vi "OCV_DMM_ApertureTime_StdDev.vi"() -> ()   [LabVIEW 2019]
panel:
  out "Error 6.5 digits AZon ADCCalon":dbl[](array[numeric])=[-1.2854850467647339e-05, -7.886710542415187e-06, 8.316335529112706e-06, 6.3393632019348445e-06, 8.358046865719615e-06] format="%#_7p"
  in  "mean values of channels 6.5 digits AZon ADCcal on":dbl[](array[numeric])=[3.4860065278089722, 3.48375553663424, 3.4808778023254034, 3.484652928409848, 3.4829310355717924] format="%#_7p"
  in  "Mean values of channels - shorted at Pogo Pins":dbl[](array[numeric])=[-6.355978921184258e-06, 2.501900814016391e-06, 1.0081969476181121e-05, 3.7724183553781954e-06, 5.872057669979462e-06] format="%#_7p"
  out "Error 100ms":dbl[](array[numeric])=[-9.674542087889648e-06, -1.2342180970570382e-06, 1.8209219958098544e-05, 4.237175472265875e-06, 4.739579464008159e-06] format="%#_7p"
  in  "Mean values of channels 100ms":dbl[](array[numeric])=[3.486009708117352, 3.4837621891266854, 3.4808876952098324, 3.4846508262221185, 3.4829274171043907] format="%#_7p"
  out "Error 83.3333ms":dbl[](array[numeric])=[-7.575016874206142e-06, -6.872566817861525e-07, 1.9622864356083625e-05, 6.5984626940185365e-06, 4.496907730189292e-06] format="%#_7p"
  in  "Mean values of channels 83.333ms":dbl[](array[numeric])=[3.4860118076425657, 3.4837627360881007, 3.4808891088542304, 3.4846531875093403, 3.482927174432657] format="%#_7p"
  out "Error 66.6666ms":dbl[](array[numeric])=[-9.609345659189472e-06, -2.0157464732939445e-06, 1.7317177337439205e-05, 4.952653229306492e-06, 4.43857256948732e-06] format="%#_7p"
  in  "Mean values of channels 66.666ms":dbl[](array[numeric])=[3.4860097733137807, 3.483761407598309, 3.4808868031672118, 3.4846515416998756, 3.482927116097496] format="%#_7p"
  out "Error 50ms":dbl[](array[numeric])=[-9.493969597151874e-06, -1.1936376171917118e-06, 1.7657588552655312e-05, 4.130477512909181e-06, 4.090088825403626e-06] format="%#_7p"
  in  "Mean values of channels 50ms":dbl[](array[numeric])=[3.4860098886898427, 3.4837622297071653, 3.480887143578427, 3.484650719524159, 3.482926767613752] format="%#_7p"
  out "Error 33.3333ms":dbl[](array[numeric])=[-9.17710259651372e-06, -2.6768859844317205e-06, 1.6583768505107344e-05, 4.873448069098174e-06, 3.1290639057601766e-06] format="%#_7p"
  in  "Mean values of channels 33.3333ms":dbl[](array[numeric])=[3.4860102055568434, 3.483760746458798, 3.4808860697583794, 3.4846514624947154, 3.4829258065888324] format="%#_7p"
  out "Error 16.6666ms":dbl[](array[numeric])=[-9.674542087889648e-06, -1.2342180970570382e-06, 1.8209219958098544e-05, 4.237175472265875e-06, 4.739579464008159e-06] format="%#_7p"
  in  "Mean values of channels 7.5 digits manual":dbl[](array[numeric])=[3.48601938265944, 3.4837634233447825, 3.4808694859898743, 3.4846465890466463, 3.4829226775249267] format="%#_7p"
  in  "Mean values of channels 16.6666ms":dbl[](array[numeric])=[3.486009708117352, 3.4837621891266854, 3.4808876952098324, 3.4846508262221185, 3.4829274171043907] format="%#_7p"
  in  "4":dbl=41.179 format="%#_6p"
  in  "3":dbl=5.212e-06 format="%#_6p"
  in  "2":dbl=1.52e-06 format="%#_6p"
  in  "1":dbl=0.2 format="%#_6p"
  in  "Test Time (s)":dbl[](array[numeric])=[4.463, 7.822, 11.163, 14.513, 17.84, 21.179] format="%#_6p"
  in  "Range (V)":dbl[](array[numeric])=[8.642e-06, 1.954e-06, 2.665e-06, 1.721e-06, 2.407e-06, 2.652e-06] format="%#_6p"
  in  "Standard Deviation (V)":dbl[](array[numeric])=[2.601e-06, 4.67064e-07, 7.14041e-07, 4.0509e-07, 6.56265e-07, 6.5863e-07] format="%#_6p"
  in  "DMM Aperture Time (s)":dbl[](array[numeric])=[0.0166666, 0.033333, 0.05, 0.0666666, 0.0833333, 0.1] format="%#_6p"
  in  "DMM Resolution (Digits)":dbl[](array[numeric])=[3.5, 4.5, 5.5, 6.5, 6.5, 7.5] format="%#_6p"
  in  "Range (V) Digits":dbl[](array[numeric])=[6.9339e-05, 7.3891e-05, 2.2514e-05, 3.346e-06, 5.505e-06, 8.62e-06] format="%#_6p"
  out "Standard Deviation vs Aperture Time":T1(graph)={"Standard Deviation (Ohm)"=[0.0166666, 0.033333, 0.05, 0.0666666, 0.0833333, 0.1], "Aperture Time (s)"=[2.601e-06, 4.67064e-07, 7.14041e-07, 4.0509e-07, 6.56265e-07, 6.5863e-07]}
  in  "Test Time (s) Digits":dbl[](array[numeric])=[1.317, 1.322, 1.418, 21.181, 57.59, 227.179] format="%#_6p"
  in  "Standard Deviation (V) Digits":dbl[](array[numeric])=[1.5947e-05, 1.7401e-05, 5.913e-06, 9.48824e-07, 1.534e-06, 2.201e-06] format="%#_6p"
  in  "DMM Aperture Time (s) Digits":dbl[](array[numeric])=[2e-05, 2e-05, 0.0005, 0.1, 0.1, 0.1] format="%#_6p"
  # "1 Average, AutoZero Once, ADC Cal Off, Settle Time 1ms"
  # "1 Average, AutoZero Once, ADC Cal Off, Settle Time 1ms"
  # "1 Average, AutoZero Once, ADC Cal Off, Settle Time 1ms"
  # "1 Average, AutoZero Once, ADC Cal Off, Settle Time 0ms"
  # "1 Average, AutoZero On, ADC Cal On, Settle Time 1ms"
  # "4 Averages, AutoZero On, ADC Cal On, Settle Time 1ms"
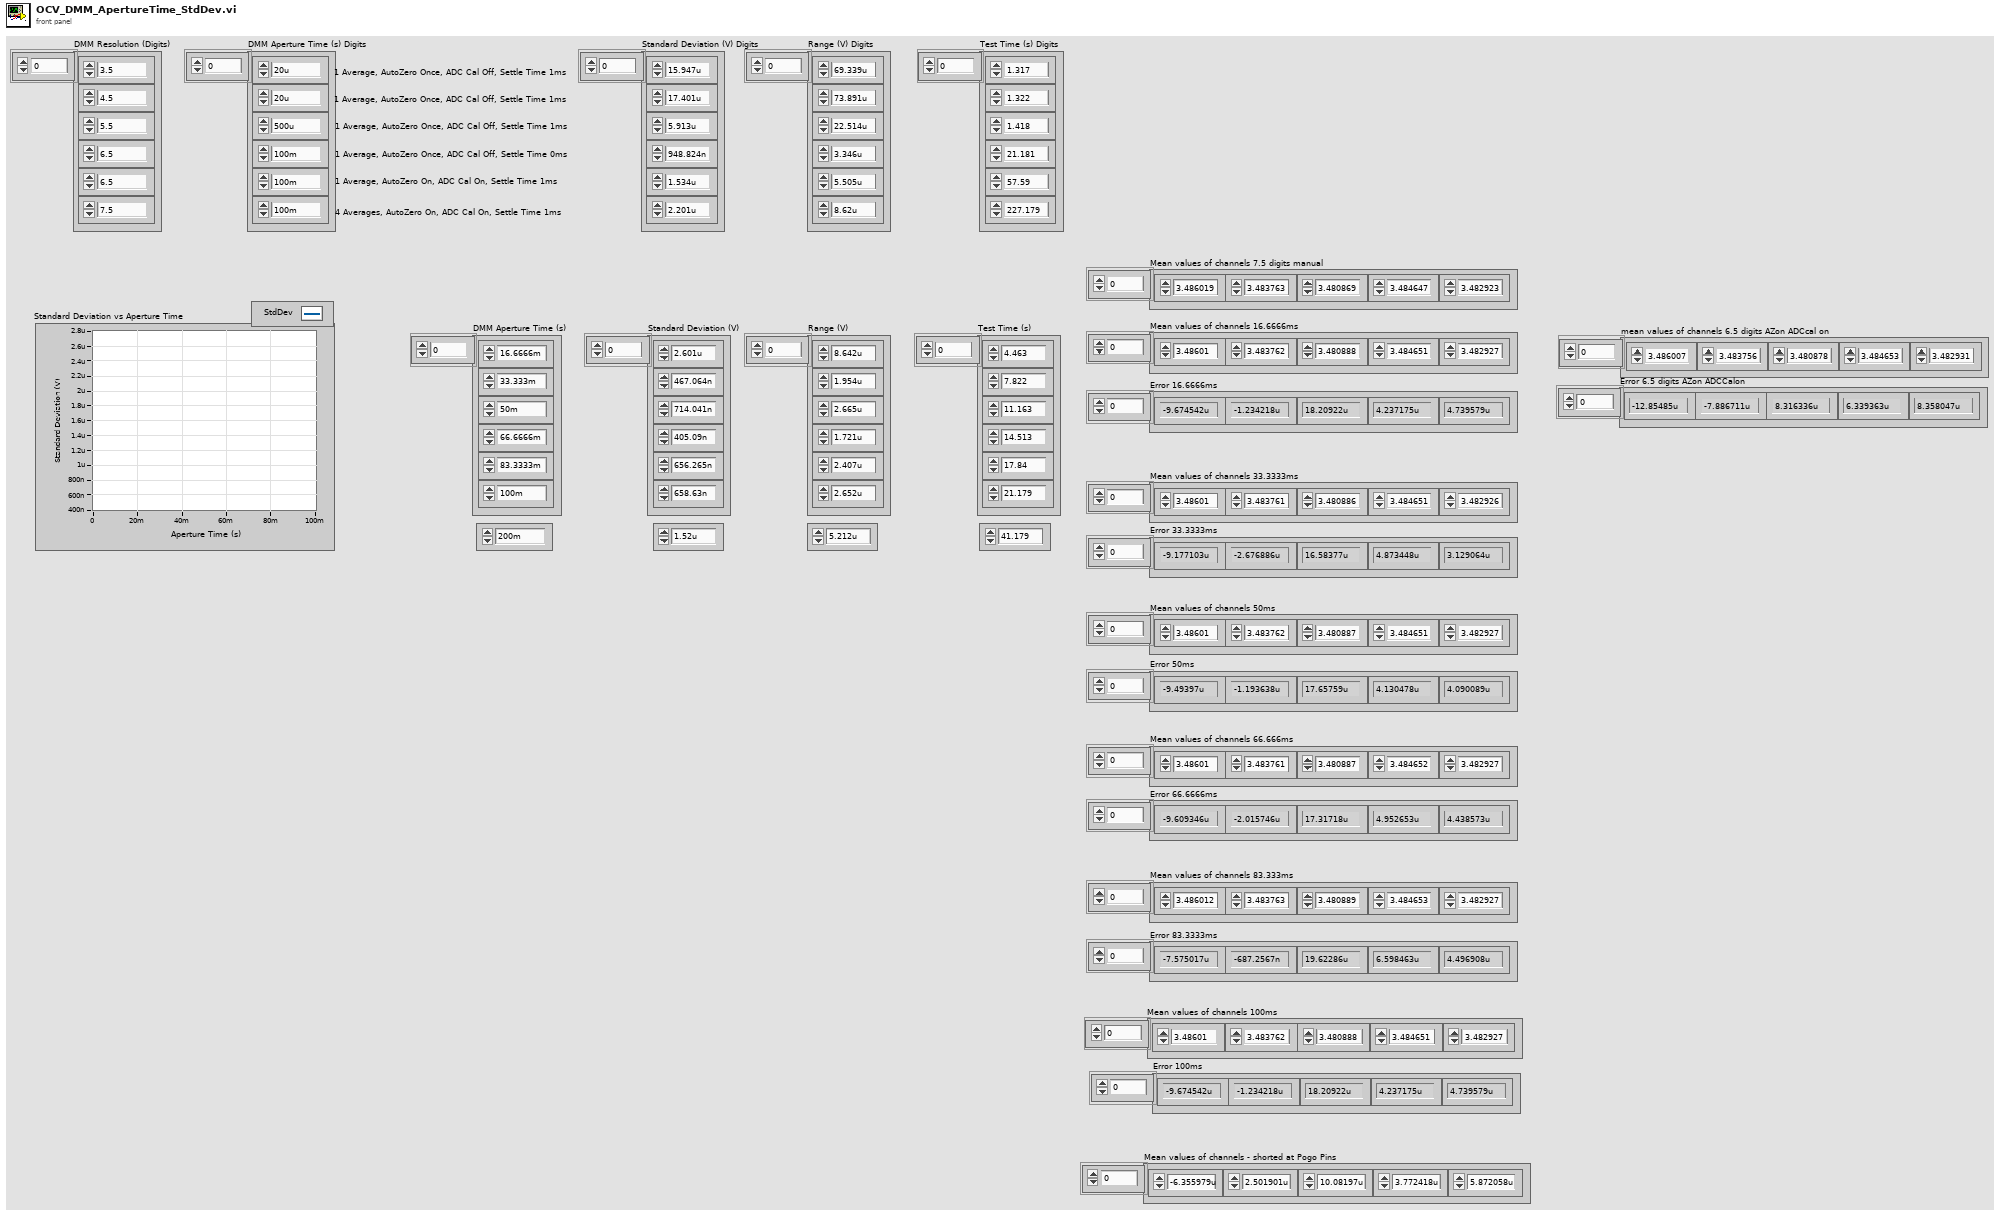
[diagram p1: front panel]
types:
  T1 = cluster{"Standard Deviation (Ohm)":dbl[], "Aperture Time (s)":dbl[]}
  T2 = cluster{"DMM Aperture Time (s)":dbl[], "Standard Deviation (V)":dbl[]}
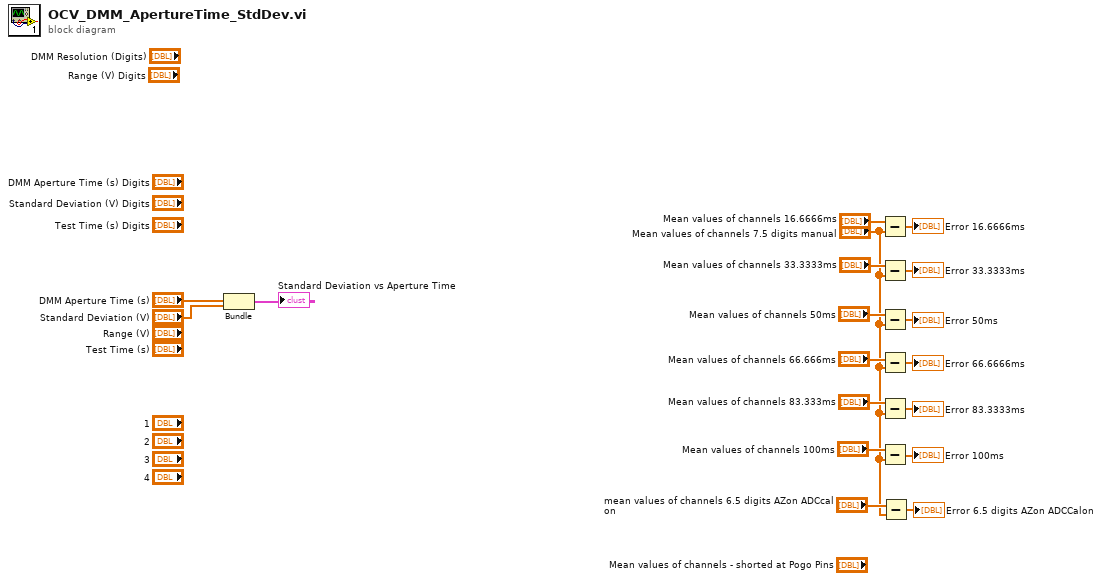
[diagram p0: block diagram]
diagram:
  n1 = Bundle("DMM Aperture Time (s)"="DMM Aperture Time (s)", "Standard Deviation (V)"="Standard Deviation (V)") -> (→"Standard Deviation vs Aperture Time":T2)  [unwired: 1 in]
  n2 = Subtract(x="Mean values of channels 16.6666ms", y="Mean values of channels 7.5 digits manual") -> (x-y=→"Error 16.6666ms":dbl[])
  n3 = Subtract(x="Mean values of channels 33.3333ms", y="Mean values of channels 7.5 digits manual") -> (x-y=→"Error 33.3333ms":dbl[])
  n4 = Subtract(x="Mean values of channels 50ms", y="Mean values of channels 7.5 digits manual") -> (x-y=→"Error 50ms":dbl[])
  n5 = Subtract(x="Mean values of channels 66.666ms", y="Mean values of channels 7.5 digits manual") -> (x-y=→"Error 66.6666ms":dbl[])
  n6 = Subtract(x="Mean values of channels 83.333ms", y="Mean values of channels 7.5 digits manual") -> (x-y=→"Error 83.3333ms":dbl[])
  n7 = Subtract(x="Mean values of channels 100ms", y="Mean values of channels 7.5 digits manual") -> (x-y=→"Error 100ms":dbl[])
  n8 = Subtract(x="mean values of channels 6.5 digits AZon ADCcal on", y="Mean values of channels 7.5 digits manual") -> (x-y=→"Error 6.5 digits AZon ADCCalon":dbl[])
